vi "Build Spec System Explorer.vi"(8 "error in (no error)":errorcluster, 9 "Action":T1) -> (0 "error out":errorcluster, 1 "Output":string)   [LabVIEW 2014, in "CD model script.lvlib"]
doc: "Constants, which are necessary for the <B>CD System Explorer LLB</B> in the generated custom device."
uses:
  CD model script.lvlib
  Constants TypDef/Build Spec System Explorer.ctl
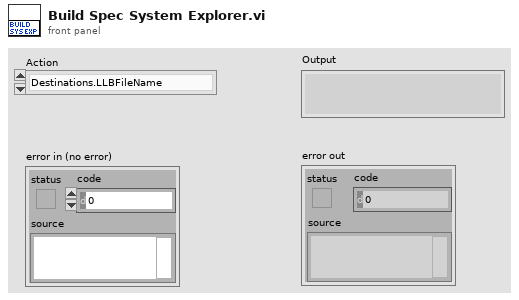
[diagram p1: front panel]
types:
  T1 = typedef "CD model script.lvlib/Build Spec System Explorer.ctl" = enum16{"Destinations.LLBFileName"}
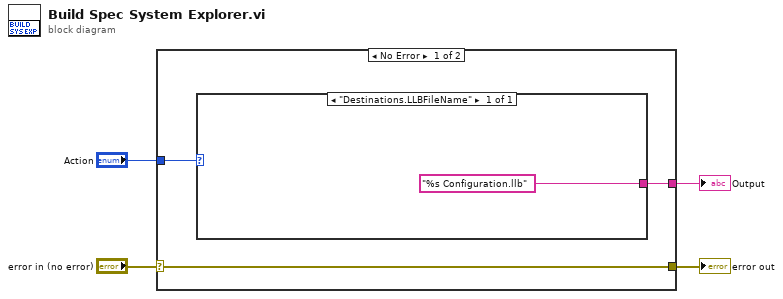
[diagram p0: block diagram]
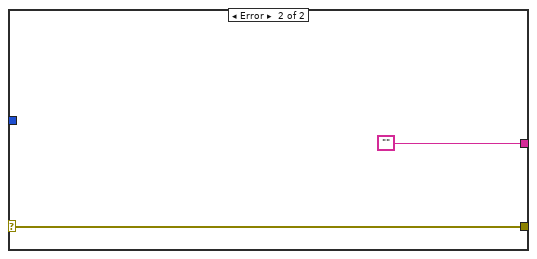
[diagram p2: hidden frame]
diagram:
  n1 = case shown="No Error" "error in (no error)" {
    selector: "error in (no error)" -> [w7 w10]
    tunnel: [w7 w10] -> w4
    tunnel: [w5 ""] -> w1
    tunnel: "Action" -> [w6 _]
    frame No Error {
      n2 = case shown="\"Destinations.LLBFileName\"" w6 {
        tunnel: ["%s Configuration.llb"] -> w5
        frame "Destinations.LLBFileName" {
        }
      }
    }
    frame Error {
    }
  }
  "error out" <- w4
  "Output" <- w1
